vi "lidarAdjust.vi"(2 "Shift type":u16(ring) items=["Shift to center", "Shift to lidar"], 3 "input":cluster{"xPos":dbl, "yPos":dbl, "Theta":dbl}={"xPos"=507.65498241430305, "yPos"=3867.916183829535, "Theta"=89.2109659500742}) -> (1 "shifted":cluster{"xPos":dbl, "yPos":dbl, "Theta":dbl}={"xPos"=507.65498241430305, "yPos"=3867.916183829535, "Theta"=89.2109659500742})   [LabVIEW 2016]
uses:
  <vilib>/Analysis/coordinate.llb/Angle Units.ctl
  <vilib>/Analysis/coordinate.llb/Angle Range (Degree).ctl
  <vilib>/Analysis/coordinate.llb/Wrap Angle (scalar).vi
  <vilib>/Analysis/NI_AAL_Angle.lvlib
panel:
  in  "distance":dbl=130.0
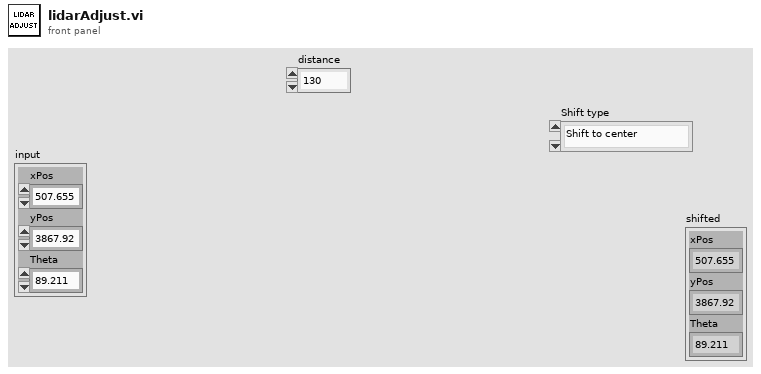
[diagram p1: front panel]
types:
  T1 = typedef "NI_AAL_Angle.lvlib/Angle Range (Degree).ctl" = u16
  T2 = typedef "NI_AAL_Angle.lvlib/Angle Units.ctl" = i32
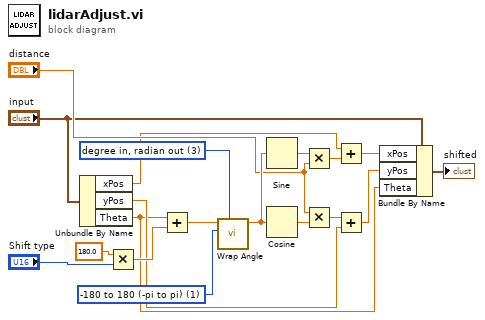
[diagram p0: block diagram]
diagram:
  w18 = T1 1 items=["none", "-180 to 180 (-pi to pi)", "0 to 360 (0 to 2pi)"] ("angle range")
  w19 = T2 3 items=["radian in, radian out", "radian in, degree out", "degree in, degree out", "degree in, radian out"] ("angle units")
  n1 = Unbundle By Name("input") -> ("xPos"=w7:dbl, "yPos"=w6:dbl, "Theta"=w3:dbl)
  n2 = Multiply(x=180.0 ("y"), y="Shift type") -> (x*y=w9:dbl)
  n3 = Add(x=w3, y=w9) -> (x+y=w11:dbl)
  n4 = call-poly <vilib>:"Wrap Angle.vi"("angle units"=w19, "angle range"=w18, "angle in"=w11) -> ("angle out"=w17:dbl)  [unwired: 7 in, 1 out]
  n5 = Sine(x=w17) -> (sin(x)=w12:dbl)
  n6 = Cosine(x=w17) -> (cos(x)=w13:dbl)
  n7 = Multiply(x=w12, y="distance") -> (x*y=w15:dbl)
  n8 = Multiply(x="distance", y=w13) -> (x*y=w14:dbl)
  n9 = Add(x=w7, y=w15) -> (x+y=w1:dbl)
  n10 = Add(x=w14, y=w6) -> (x+y=w2:dbl)
  n11 = Bundle By Name(cluster="input", "xPos"=w1, "yPos"=w2, "Theta"=w3) -> (→"shifted":cluster{"xPos":dbl, "yPos":dbl, "Theta":dbl})
